vi "mxwScript_Cmnd2Str_lockMainVI.vi"(8 "error in (no error)":errorcluster, 11 "data":variant) -> (0 "error out":errorcluster, 3 "outputString":string)   [LabVIEW 2017]
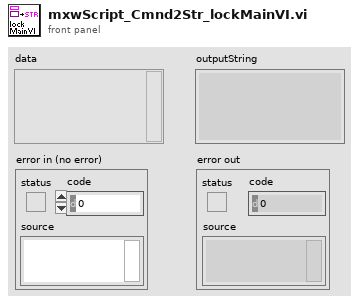
[diagram p1: front panel]
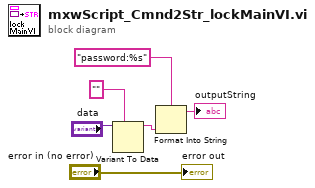
[diagram p0: block diagram]
diagram:
  n1 = Variant To Data(type="", Variant="data") -> (data=w1:string)  [unwired: 1 in, 1 out]
  n2 = Format Into String(format string="password:%s", w1) -> (resulting string=→"outputString":string)  [unwired: 2 in, 1 out]
  "error out" <- "error in (no error)"
